vi "update name.vi"(8 "error in (no error)":errorcluster, 10 "Desired Alias":string="Modbus ", 11 "Parent Ref in":T1=18446744073709551615 format="%.0x") -> (0 "error out":errorcluster, 3 "Parent Ref dup":T1=18446744073709551615 format="%.0x")   [LabVIEW 2021, in "Modbus Master System Explorer.lvlib"]
uses:
  Modbus Master System Explorer.lvlib
  <vilib>/NI VeriStand/Custom Device API/Custom Device Item Ref.ctl
  <vilib>/NI VeriStand/Custom Device Tools/Custom Device Utility Library/Custom Device Utility Library.lvlib
  <vilib>/NI VeriStand/Custom Device API/Custom Device API.lvlib
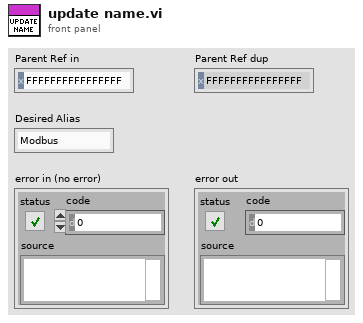
[diagram p1: front panel]
types:
  T1 = typedef "Custom Device API.lvlib/Custom Device Item Ref.ctl" = u64
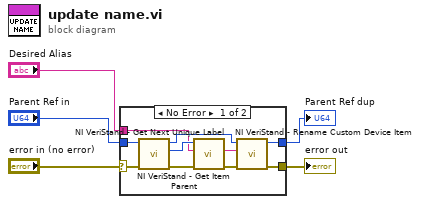
[diagram p0: block diagram]
diagram:
  n1 = case shown="No Error" "error in (no error)" {
    selector: "error in (no error)" -> [w7 w16]
    tunnel: [w15 w16] -> w5
    tunnel: [w14 w17] -> w4
    tunnel: "Parent Ref in" -> [w12 w17]
    tunnel: "Desired Alias" -> [w9 _]
    frame No Error {
      n2 = call <vilib>:"NI VeriStand - Get Item Parent.vi"("error in (no error)"=w7, "Item Ref in"=w12) -> ("error out"=w6:errorcluster, "Parent Ref"=w11:T1, "Item Ref out"=w10:T1)  [unwired: 6 in, 1 out]
      n3 = call <vilib>:"NI VeriStand - Get Next Unique Label.vi"("error in (no error)"=w6, "Label"=w9, "Parent Ref in"=w11) -> ("error out"=w13:errorcluster, "Label out"=w8:string)  [unwired: 5 in, 2 out]
      n4 = call <vilib>:"NI VeriStand - Rename Custom Device Item.vi"("error in (no error)"=w13, "New Name"=w8, "Item Ref in"=w10) -> ("error out"=w15:errorcluster, "Item Ref out"=w14:T1)  [unwired: 1 in, 6 out]
    }
    frame Error {
    }
  }
  "error out" <- w5
  "Parent Ref dup" <- w4
